vi "MB Ethernet Example Slave.vi"() -> ()   [LabVIEW 2023, in "Voegtlin_NI_SMART_Modbus_Drivers.lvlib"]
uses:
  Voegtlin_NI_SMART_Modbus_Drivers.lvlib
  MB Slave Init (poly).vi
  MB Globals.vi
  MB Slave Read All Coils (poly).vi
  MB Slave Read All Holding Registers (poly).vi
  MB Slave Write Input Registers (poly).vi
  MB Slave Write Discrete Inputs (poly).vi
panel:
  in  "Discrete Inputs (Master can only read these)":bool[](array[boolean])=[FALSE, FALSE, FALSE, FALSE]
  in  "Input Registers (Master can only read these)":u16[](array[numeric])=[0, 0, 0, 0]
  in  "Listening Port":u16=502
  in  "Stop":bool
  out "Holding Registers":u16[](array[numeric]) caption="Holding Registers (Master can write in these registers)"
  out "Coils":bool[](array[boolean]) caption="Coils (Master can write coils)"
  # "MB Ethernet Example Slave.vi\n\nInstructions\n1. Run this VI first (Slave/Server)\n2. Open and run MB Ethernet Example Master.vi\n3. Modify the discrete inputs or input registers on the slave -> they're updated on the master.\n4. Modify the coils and registers on the master -> they're updated on the slave."
  # "TCP Settings"
  # "Slave Registers"
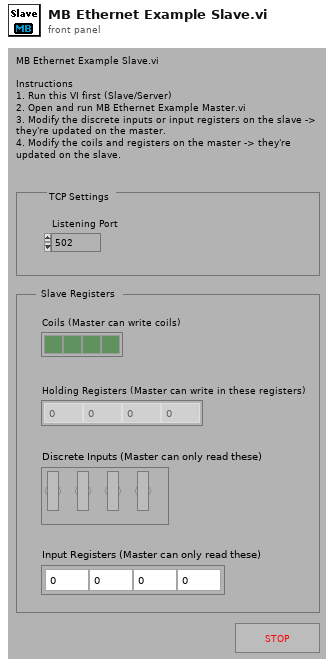
[diagram p1: front panel]
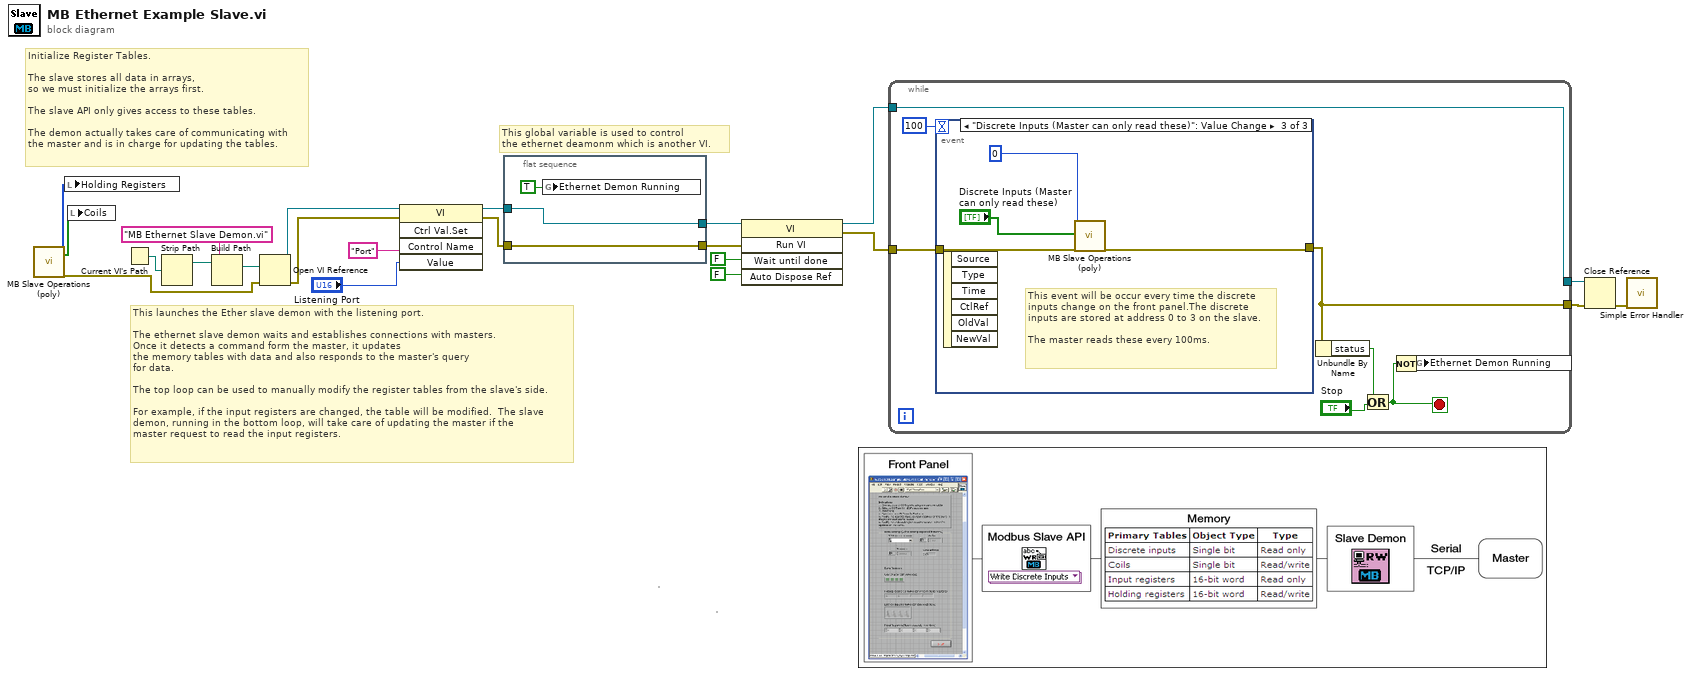
[diagram p0: block diagram]
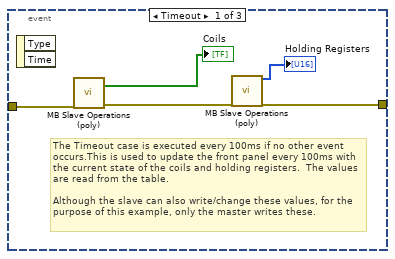
[diagram p2: hidden frame]
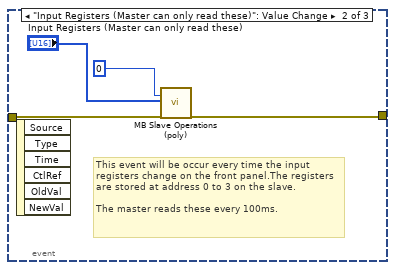
[diagram p3: hidden frame]
diagram:
  # "This global variable is used to control\nthe ethernet deamonm which is another VI."
  # "Initialize Register Tables.\n\nThe slave stores all data in arrays,\nso we must initialize the arrays first.  \n\nThe slave API only gives access to these tables. \n\nThe demon actually takes care of communicating with \nthe master and is in charge for updating the tables."
  # "This launches the Ether slave demon with the listening port.\n\nThe ethernet slave demon waits and establishes connections with masters.  \nOnce it detects a command form the master, it updates\nthe memory tables with data and also responds to the master's query\nfor data.\n\nThe top loop can be used to manually modify the register tables from the slave's side.\n\nFor example, if the input registers are changed, the table will be modified.  The slave\ndemon, running in the bottom loop, will take care of updating the master if the \nmaster request to read the input registers."
  n1 = call-poly "MB Slave Operations (poly).vi"() -> ("Holding Registers"=w22:u16[], "Coils"=w5:bool[], "error out"=w8:errorcluster)  [unwired: 1 in, 16 out]
  n2 = local write "Holding Registers"(w22) -> ()
  n3 = local write "Coils"(w5) -> ()
  n4 = Current VI's Path() -> (path=w18:path)
  n5 = Strip Path(path=w18) -> (stripped path=w19:path)  [unwired: 1 out]
  n6 = Build Path(base path=w19, name or relative path="MB Ethernet Slave Demon.vi") -> (appended path=w21:path)
  n7 = Open VI Reference(vi path=w21, error in (no error)=w8) -> (vi reference=w15:refnum<vi>, error out=w14:errorcluster)  [unwired: 4 out]
  n8 = invoke class="VI" method="Ctrl Val.Set"(reference=w15, error in=w14, "Control Name"="Port", "Value"="Listening Port") -> (reference out=w1:refnum<vi>, error out=w2:errorcluster)  [unwired: 1 in, 3 out]
  n9 = flat-sequence {
    tunnel: [w25] -> w7
    tunnel: w2 -> [w25]
    tunnel: [w23] -> w4
    tunnel: w1 -> [w23]
    frame #0 {
      n10 = global write "MB Globals.vi" "Ethernet Demon Running"(TRUE ("Slave Demon Running")) -> ()
    }
  }
  n11 = invoke class="VI" method="Run VI"(reference=w4, error in=w7, "Wait until done"=FALSE, "Auto Dispose Ref"=FALSE) -> (reference out=w10:refnum<vi>, error out=w6:errorcluster)  [unwired: 1 in, 3 out]
  n12 = while {
    tunnel: [w28] -> w11
    tunnel: w10 -> [w28]
    tunnel: [w27] -> w9
    tunnel: w6 -> [w26]
    stop <- w29 stop-if-true
    n13 = event shown="[2] \"Discrete Inputs (Master can only read these)\": Value Change" {
      selector: _ -> [_ _ _]
      dyn-events: _ -> [_ _ _]
      timeout: 100 -> [_ _ _]
      tunnel: w26 -> [w38 w42 w46]
      tunnel: [w35 w40 w44] -> w27
      event Timeout {
        # "The Timeout case is executed every 100ms if no other event occurs.This is used to update the front panel every 100ms with the current state of the coils and holding registers.  The values are read from the table. \n\nAlthough the slave can also write/change these values, for the purpose of this example, only the master writes these."
        n14 = event-data() -> ()  [unwired: 3 out]
        n15 = call-poly "MB Slave Operations (poly).vi"("error in"=w38) -> ("Coils"=→"Coils":bool[], "error out"=w36:errorcluster)  [unwired: 17 out]
        n16 = call-poly "MB Slave Operations (poly).vi"("error in"=w36) -> ("Holding Registers"=→"Holding Registers":u16[], "error out"=w35:errorcluster)  [unwired: 17 out]
      }
      event "Input Registers (Master can only read these)": Value Change {
        # "This event will be occur every time the input registers change on the front panel.The registers are stored at address 0 to 3 on the slave.\n \nThe master reads these every 100ms."
        n17 = event-data() -> ()  [unwired: 7 out]
        n18 = call-poly "MB Slave Operations (poly).vi"("Starting Address"=u16 0 ("Address"), "Input Registers"="Input Registers (Master can only read these)", "error in"=w42) -> ("error out"=w40:errorcluster)  [unwired: 1 in, 15 out]
      }
      event "Discrete Inputs (Master can only read these)": Value Change {
        # "This event will be occur every time the discrete inputs change on the front panel.The discrete inputs are stored at address 0 to 3 on the slave.\n \nThe master reads these every 100ms."
        n19 = event-data() -> ()  [unwired: 7 out]
        n20 = call-poly "MB Slave Operations (poly).vi"("Starting Address"=u16 0, "Discrete Inputs"="Discrete Inputs (Master can only read these)", "error in"=w46) -> ("error out"=w44:errorcluster)  [unwired: 1 in, 15 out]
      }
    }
    n21 = Unbundle By Name(w27) -> ("status"=w32:bool)
    n22 = Or(x=w32, y="Stop") -> (x .or. y?=w29:bool)
    n23 = Not(x=w29) -> (.not. x?=w30:bool)
    n24 = global write "MB Globals.vi" "Ethernet Demon Running"(w30) -> ()
  }
  n25 = Close Reference(reference=w11, error in (no error)=w9) -> (error out=w3:errorcluster)
  n26 = call <vilib>:"Simple Error Handler.vi"("error in (no error)"=w3) -> ()  [unwired: 1 in, 8 out]
